vi "Write ExposureTime.vi"(8 "error in (no error)":errorcluster, 10 "ExposureTime [ms]":i32, 11 "CCD in":refnum<class "CCD.lvclass">) -> (0 "error out":errorcluster, 3 "CCD out":refnum<class "CCD.lvclass">)   [LabVIEW 2023, in "CCD.lvclass"]
uses:
  CCD.lvclass
  CCD.lvclass/CCD.ctl
  b16bc14f-8648-4bf2-89fe-13759e9f46f2.vi
  Libraries/DeviceManager/DeviceManager.lvlib
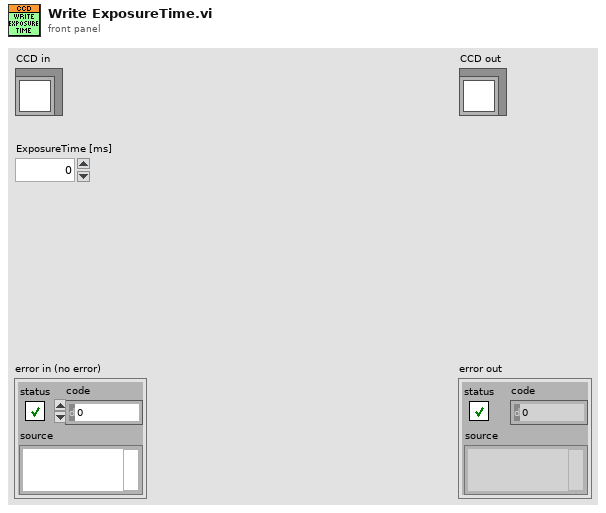
[diagram p1: front panel]
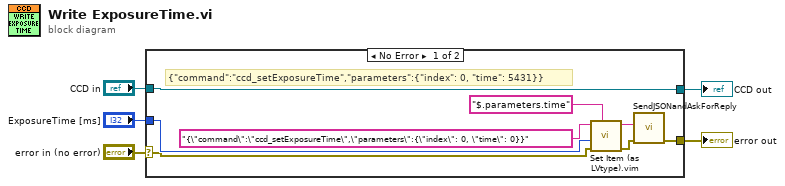
[diagram p0: block diagram]
diagram:
  n1 = case shown="No Error" "error in (no error)" {
    selector: "error in (no error)" -> [w7 w14]
    tunnel: [w6 w14] -> w4
    tunnel: [w13 w15] -> w2
    tunnel: "CCD in" -> [w13 w15]
    tunnel: "ExposureTime [ms]" -> [w10 _]
    frame No Error {
      # "{\"command\":\"ccd_setExposureTime\",\"parameters\":{\"index\": 0, \"time\": 5431}}"
      n2 = call "Set Item (as LVtype).vim"("$Path or Item Name"="$.parameters.time", "error in (no error)"=w7, "Anything"=w10, "JSON"="{\"command\":\"ccd_setExposureTime\",\"parameters\":{\"index\": 0, \"time\": 0}}") -> ("error out"=w8:errorcluster, "<JSON>"=w9:string)  [unwired: 4 in, 1 out]
      n3 = call "SendJSONandAskForReply.vi"("error in"=w8, "JSON to be sent"=w9) -> ("error out"=w6:errorcluster)  [unwired: 7 in, 2 out]
    }
    frame Error {
    }
  }
  "error out" <- w4
  "CCD out" <- w2
